vi "GetTagByCoords__slk_mt.vi"(8 "error in (no error)":errorcluster, 10 "coordinates":cluster{"Horizontal":i32, "Vertical":i32}, 11 "tree view in":refnum<class "TreeView__slk_mt.lvclass">) -> (0 "error out":errorcluster, 2 "tag":string, 3 "tree view out":refnum<class "TreeView__slk_mt.lvclass">)   [LabVIEW 2020, in "Lazyboots Menu Tool.lvlib" / "TreeView__slk_mt.lvclass"]
doc: "Returns a tag with specified coordinate."
uses:
  TreeView__slk_mt.lvclass
  TreeView__slk_mt.lvclass/TreeView__slk_mt.ctl
panel:
  # "GetTagByCoords__slk_mt.vi\nReturns a tag with specified coordinate.\n\nNOTICE -- YOU MUST LEAVE THIS NOTICE IN PLACE.\n\nCopyright (c) 2011, LIANG LIU Shawn.Liu.cn@gmail.com\nAll rights reserved.\n\nRedistribution and use in source and binary forms, with or without modification, are permitted provided that the following conditions are met:\n-Redistributions of source code must retain the above copyright notice, this list of conditions and the following disclaimer.\n-Redistributions in binary form must reproduce the above copyright notice, this list of conditions and the following disclaimer in the documentation and/or other materials provided with the distribution.\n-Neither the name of the eLp nor the names of its contributors may be used to endorse or promote products derived from this software without specific prior written permission.\n\nTHIS SOFTWARE IS PROVIDED BY THE COPYRIGHT HOLDERS AND CONTRIBUTORS \"AS IS\" AND ANY EXPRESS OR IMPLIED WARRANTIES, INCLUDING, BUT NOT LIMITED TO, THE IMPLIED WARRANTIES OF MERCHANTABILITY AND FITNESS FOR A PARTICULAR PURPOSE ARE DISCLAIMED. IN NO EVENT SHALL THE COPYRIGHT HOLDER OR CONTRIBUTORS BE LIABLE FOR ANY DIRECT, INDIRECT, INCIDENTAL, SPECIAL, EXEMPLARY, OR CONSEQUENTIAL DAMAGES (INCLUDING, BUT NOT LIMITED TO, PROCUREMENT OF SUBSTITUTE GOODS OR SERVICES; LOSS OF USE, DATA, OR PROFITS; OR BUSINESS INTERRUPTION) HOWEVER CAUSED AND ON ANY THEORY OF LIABILITY, WHETHER IN CONTRACT, STRICT LIABILITY, OR TORT (INCLUDING NEGLIGENCE OR OTHERWISE) ARISING IN ANY WAY OUT OF THE USE OF THIS SOFTWARE, EVEN IF ADVISED OF THE POSSIBILITY OF SUCH DAMAGE."
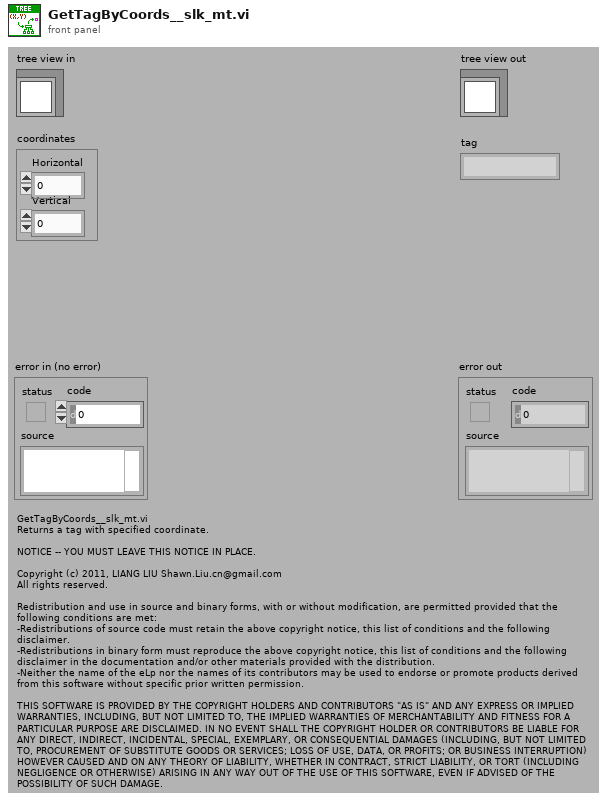
[diagram p1: front panel]
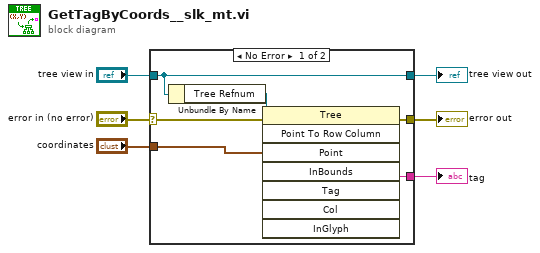
[diagram p0: block diagram]
diagram:
  n1 = case shown="No Error" "error in (no error)" {
    selector: "error in (no error)" -> [w10 w14]
    tunnel: [w9 w14] -> w5
    tunnel: [w11 w13] -> w3
    tunnel: "tree view in" -> [w11 w13]
    tunnel: "coordinates" -> [w7 _]
    tunnel: [w8 _] -> w2
    frame No Error {
      n2 = Unbundle By Name(w11) -> ("Tree Refnum"=w12:refnum<vi>)
      n3 = invoke class="Tree" method="Point To Row Column"(reference=w12, error in=w10, "Point"=w7) -> (error out=w9:errorcluster, "Tag"=w8:string)  [unwired: 5 in, 6 out]
    }
    frame Error {
    }
  }
  "error out" <- w5
  "tree view out" <- w3
  "tag" <- w2
